vi "ytscanboxB.vi"(4 "Color FG":u32(colorbox)=6416282, 6 "Poztion":T1(ring)=enum."中", 7 "YTESTER测试数据":T2={"Socket(From1)"=1, "SN"=refnum, "StopFlagRef"=refnum, "YT System Queue"=refnum}, 8 "类回车确认":bool=TRUE, 9 "扫码项开头匹配":string, 10 "扫码长度":i32, 11 "扫码项名称":string="SN：") -> (0 "pass?":bool, 3 "SN out":string)   [LabVIEW 2017]
doc: "yyll"
uses:
  YtCommon.lvlibp/yt`Step TestData.ctl
  YtCommon.lvlibp/yt`Step System Queue.ctl
  <vilib>/Utility/miscctls.llb/LVPointTypeDef.ctl
  <vilib>/event_ctls.llb/eventvkey.ctl
  YtCommon.lvlibp
panel:
  in  "check":bool=TRUE
  in  "SN":string caption="SN： [长度0][需回车]"
  # "YYLL.ScanBoxB"
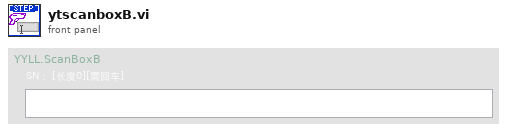
[diagram p1: front panel]
types:
  T1 = enum16{"↖", "↑", "↗", "←", "中", "→", "↙", "↓", "↘"}
  T2 = typedef "YtCommon.lvlibp/yt`Step TestData.ctl" = cluster{"Socket(From1)":i32, "SN":refnum<notifier>, "StopFlagRef":refnum<notifier>, "YT System Queue":refnum<queue>}
  T3 = typedef "LVPointTypeDef.ctl" = cluster{"Horizontal":i16, "Vertical":i16}
  T4 = typedef "eventvkey.ctl" = enum16{"ASCII", "Enter", "Return", "Shift", "Ctrl", "Alt", "Cmd", "Opt", "Caps", "NumLock", "Clear", "Break", "Up", "Down", "Left", "Right", "Insert", "Delete", "Home", "End", "PageUp", "PageDown", "Escape", "Help", "Pause", "ScrollLock", "F1", "F2", "F3", "F4", "F5", "F6", "F7", "F8", "F9", "F10", "F11", "F12", "F13", "F14", "F15", "F16", "F17", "F18", "F19", "F20", "F21", "F22", "F23", "F24", "Play", "VolumeUp", "VolumeDown", "Mute", "Two Byte Char"}
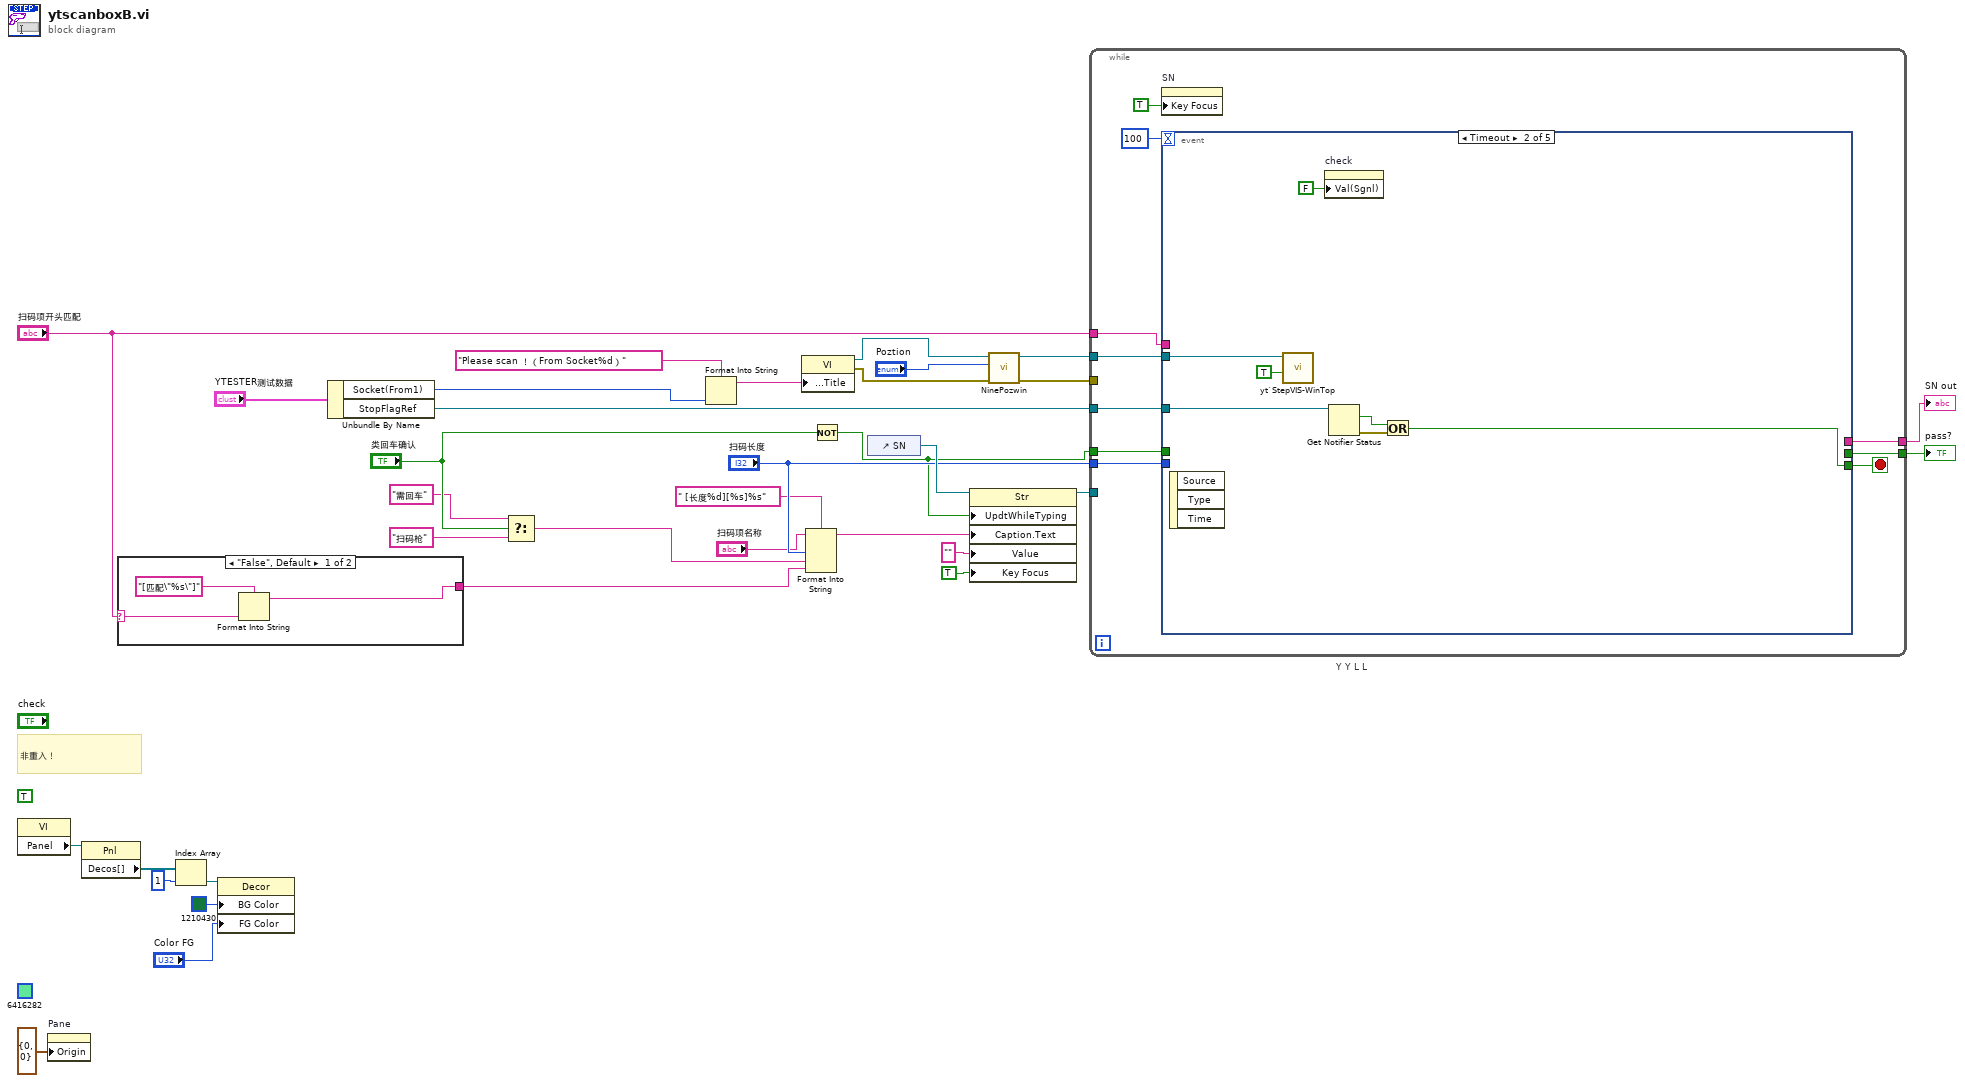
[diagram p0: block diagram]
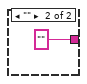
[diagram p2: hidden frame]
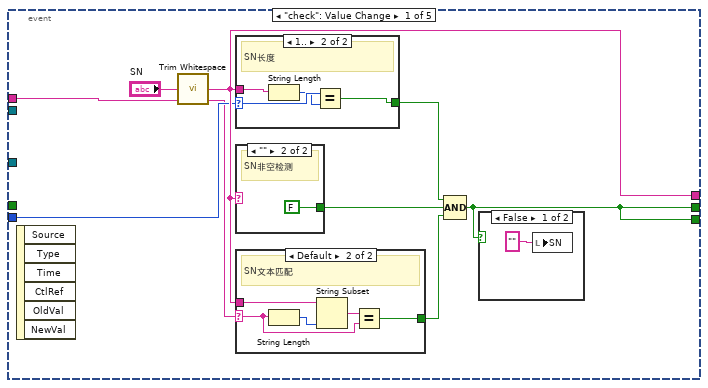
[diagram p3: hidden frame]
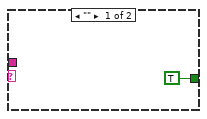
[diagram p5: hidden frame]
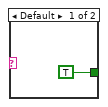
[diagram p6: hidden frame]
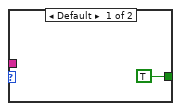
[diagram p7: hidden frame]
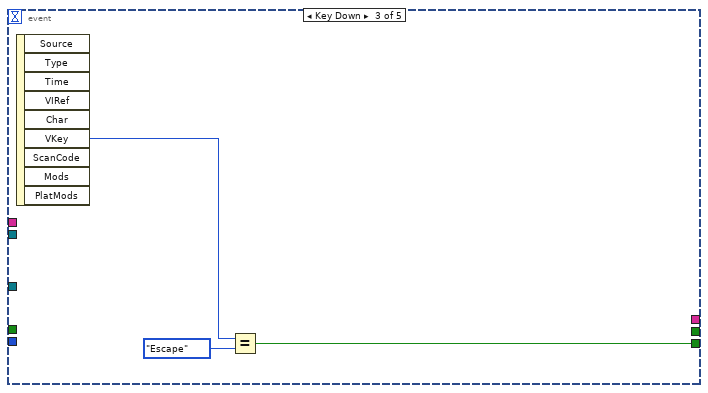
[diagram p8: hidden frame]
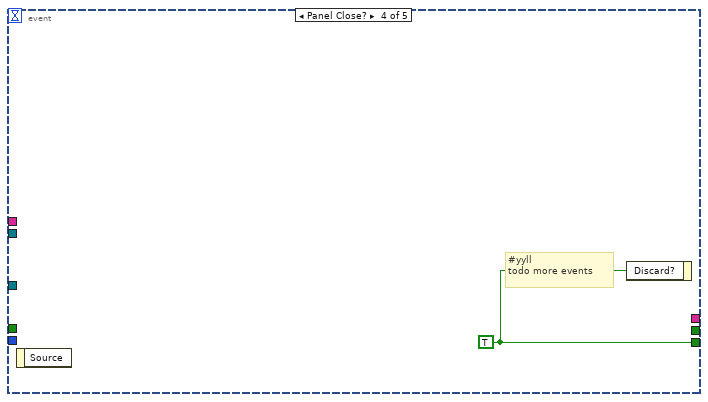
[diagram p9: hidden frame]
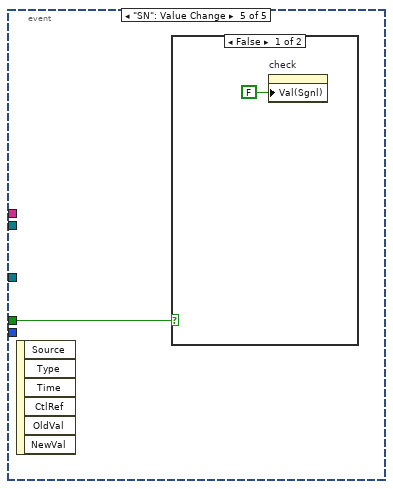
[diagram p10: hidden frame]
diagram:
  (unwired) u32 6416282 ("Color Box 2")
  (unwired) TRUE
  # "非重入！"
  # "Y Y L L"
  n1 = property class="VI"() -> ("Panel"=w23:refnum<vi>)  [unwired: 2 in, 2 out]
  n2 = property on="Pane" class="Pane"("Origin"=T3 {"Horizontal"=0, "Vertical"=0}) -> ()  [unwired: 2 in, 2 out]
  n3 = property class="Pnl"(reference=w23) -> ("Decos[]"=w22:refnum<vi>[])  [unwired: 1 in, 2 out]
  n4 = case shown="\"False\", Default" "扫码项开头匹配" {
    selector: "扫码项开头匹配" -> [w37 _]
    tunnel: [w36 ""] -> w6
    frame "False", Default {
      n5 = Format Into String(format string="[匹配\"%s\"]", w37) -> (resulting string=w36:string)  [unwired: 2 in, 1 out]
    }
    frame "" {
    }
  }
  n6 = Index Array(array=w22, index=1) -> (element=w21:refnum<vi>)
  n7 = property class="Decor"(reference=w21, "BG Color"=u32 1210430 ("Color Box"), "FG Color"="Color FG") -> ()  [unwired: 1 in, 2 out]
  n8 = Unbundle By Name("YTESTER测试数据") -> ("Socket(From1)"=w25:i32, "StopFlagRef"=w27:refnum<notifier>)
  n9 = Select(t="需回车" ("format string"), s="类回车确认", f="扫码枪" ("format string")) -> (s? t:f=w8:string)
  n10 = Format Into String(format string="Please scan ！（From Socket%d）", w25) -> (resulting string=w24:string)  [unwired: 2 in, 1 out]
  n11 = property class="VI"("Front Panel.Title"=w24) -> (reference out=w5:refnum<vi>, error out=w2:errorcluster)  [unwired: 2 in]
  n12 = Format Into String(format string=" [长度%d][%s]%s", initial string="扫码项名称", "扫码长度", w8, w6) -> (resulting string=w14:string)  [unwired: 1 in, 1 out]
  n13 = Not(x="类回车确认") -> (.not. x?=w12:bool)
  n14 = control-ref of="SN"() -> (w32:refnum<vi>)
  n15 = property class="Str"(reference=w32, "UpdtWhileTyping"=w12, "Caption.Text"=w14, "Value"="", "Key Focus"=TRUE) -> (reference out=w29:refnum<vi>)  [unwired: 1 in, 1 out]
  n16 = call "NinePozwin.vi"("error in (no error)"=w2, "Poztion"="Poztion", "VI ref"=w5) -> ("error out"=w4:errorcluster, "reference out"=w1:refnum<vi>)  [unwired: 7 in]
  n17 = while {
    tunnel: [w46] -> w34
    tunnel: w29 -> [_]
    tunnel: w27 -> [w45]
    tunnel: "扫码长度" -> [w44]
    tunnel: [w43] -> w13
    tunnel: w12 -> [w41]
    tunnel: "扫码项开头匹配" -> [w40]
    tunnel: w4 -> [_]
    tunnel: w1 -> [w39]
    stop <- w47 stop-if-true
    n18 = property on="SN" class="Str"("Key Focus"=TRUE) -> ()  [unwired: 2 in, 2 out]
    n19 = event shown="[1] Timeout" {
      selector: _ -> [_ _ _ _ _]
      dyn-events: _ -> [_ _ _ _ _]
      timeout: 100 -> [_ _ _ _ _]
      tunnel: [w50 w73 w78 w81 _] -> w47
      tunnel: [w53 _ _ _ _] -> w46
      tunnel: w45 -> [_ w76 _ _ _]
      tunnel: w44 -> [w51 _ _ _ _]
      tunnel: [w50 _ _ _ _] -> w43
      tunnel: w41 -> [_ _ _ _ w82]
      tunnel: w40 -> [w49 _ _ _ _]
      tunnel: w39 -> [_ w71 _ _ _]
      event "check": Value Change {
        n20 = event-data() -> ()  [unwired: 1 in, 6 out]
        n21 = call <vilib>:"Trim Whitespace.vi"("string"="SN") -> ("trimmed string"=w53:string)  [unwired: 1 in]
        n22 = case shown="1.." w51 {
          selector: w51 -> [_ w69]
          tunnel: w53 -> [_ w70]
          tunnel: [TRUE w67] -> w56
          frame Default {
          }
          frame 1.. {
            # "SN长度"
            n23 = String Length(string=w70) -> (length=w68:i32)
            n24 = Equal?(x=w69, y=w68) -> (x = y?=w67:bool)
          }
        }
        n25 = case shown="\"\"" w53 {
          tunnel: [TRUE FALSE] -> w55
          frame Default {
          }
          frame "" {
            # "SN非空检测"
          }
        }
        n26 = case shown="Default" w49 {
          selector: w49 -> [_ w62]
          tunnel: [TRUE w61] -> w54
          tunnel: w53 -> [_ w63]
          frame "" {
          }
          frame Default {
            # "SN文本匹配"
            n27 = String Length(string=w62) -> (length=w60:i32)
            n28 = String Subset(string=w63, length (rest)=w60) -> (substring=w59:string)  [unwired: 1 in]
            n29 = Equal?(x=w59, y=w62) -> (x = y?=w61:bool)
          }
        }
        n30 = Compound Arithmetic op=AND(w56, w55, w54) -> (w50:bool)
        n31 = case shown="False" w50 {
          frame False {
            n32 = local write "SN"("" ("SN")) -> ()
          }
          frame True {
          }
        }
      }
      event Timeout {
        n33 = event-data() -> ()  [unwired: 1 in, 3 out]
        n34 = call "yt`StepVIS-WinTop.vi"("一直置顶？（F）"=TRUE, "vi ref（TopVIs）"=w71) -> ()  [unwired: 9 in, 1 out]
        n35 = property on="check" class="Bool (strict)"("Val(Sgnl)"=FALSE ("Value (Signaling)")) -> ()  [unwired: 2 in, 2 out]
        n36 = Get Notifier Status(notifier=w76) -> (current notification=w75:bool, error out=w74:errorcluster)  [unwired: 1 in, 3 out]
        n37 = Or(x=w75, y=w74) -> (x .or. y?=w73:bool)
      }
      event Key Down {
        n38 = event-data() -> ("VKey"=w80:T4)  [unwired: 1 in, 8 out]
        n39 = Equal?(x=w80, y=eventvkey."Escape" ("VKey")) -> (x = y?=w78:bool)
      }
      event Panel Close? {
        w81 = TRUE ("Discard?")
        # "#yyll\ntodo more events"
        n40 = event-data() -> ()  [unwired: 1 in, 1 out]
        n41 = event-data("Discard?"=w81) -> ()  [unwired: 1 in, 1 out]
      }
      event "SN": Value Change {
        n42 = event-data() -> ()  [unwired: 1 in, 6 out]
        n43 = case shown="False" w82 {
          frame False {
            n44 = property on="check" class="Bool (strict)"("Val(Sgnl)"=FALSE ("Value (Signaling)")) -> ()  [unwired: 2 in, 2 out]
          }
          frame True {
          }
        }
      }
    }
  }
  "SN out" <- w34
  "pass?" <- w13
